vi "replace AO XYwfparam.vi"(0 "Baseline (V)":dbl, 1 "Start amplitude (V)":dbl, 2 "Cycles":dbl, 3 "Repeats":dbl, 4 "index of AO wave":i32, 5 "Step size (V)":dbl, 7 "DC (%)":dbl, 9 "Sampling frequency (Hz)":dbl, 11 "Period (ms)":dbl, 12 "Cycle length (s)":dbl, 13 "Pulses":dbl, 14 "padding value":dbl, 15 "Matlab wave name":path) -> ()   [LabVIEW 2015]
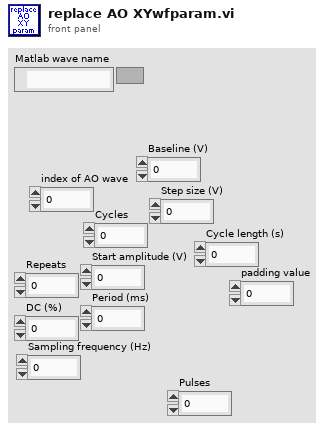
[diagram p1: front panel]
types:
  T1 = cluster{"AO parameters":cluster{"AOtab":dbl, "Repeats":dbl, "Cycles":dbl, "Start amplitude (V)":dbl, "Baseline (V)":dbl, "Step size (V)":dbl, "DC (%)":dbl, "Sampling frequency (Hz)":dbl, "Period (ms)":dbl, "Offset (V)":dbl, "Amplitude (V)":dbl, "Frequency":dbl, "Tri Repeats":dbl, "phase shift (ms)":dbl, "Pulses":dbl, "Matlab wave file":path, "Tri phase":dbl, "padding value":dbl}[], "DO parameters":cluster{"Digital DC (%)":dbl, "Digital phase":dbl, "Digital Freq (Hz)":dbl, "Sampling frequency (Hz)":dbl, "Digital time offset (s) ":dbl, "padding value":dbl, "matlab wave file":path, "DOtab":dbl}[]}
  T2 = cluster{"AOtab":dbl, "Repeats":dbl, "Cycles":dbl, "Start amplitude (V)":dbl, "Baseline (V)":dbl, "Step size (V)":dbl, "DC (%)":dbl, "Sampling frequency (Hz)":dbl, "Period (ms)":dbl, "Offset (V)":dbl, "Amplitude (V)":dbl, "Frequency":dbl, "Tri Repeats":dbl, "phase shift (ms)":dbl, "Pulses":dbl, "Matlab wave file":path, "Tri phase":dbl, "padding value":dbl}[]
  T3 = cluster{"AOtab":dbl, "Repeats":dbl, "Cycles":dbl, "Start amplitude (V)":dbl, "Baseline (V)":dbl, "Step size (V)":dbl, "DC (%)":dbl, "Sampling frequency (Hz)":dbl, "Period (ms)":dbl, "Offset (V)":dbl, "Amplitude (V)":dbl, "Frequency":dbl, "Tri Repeats":dbl, "phase shift (ms)":dbl, "Pulses":dbl, "Matlab wave file":path, "Tri phase":dbl, "padding value":dbl}
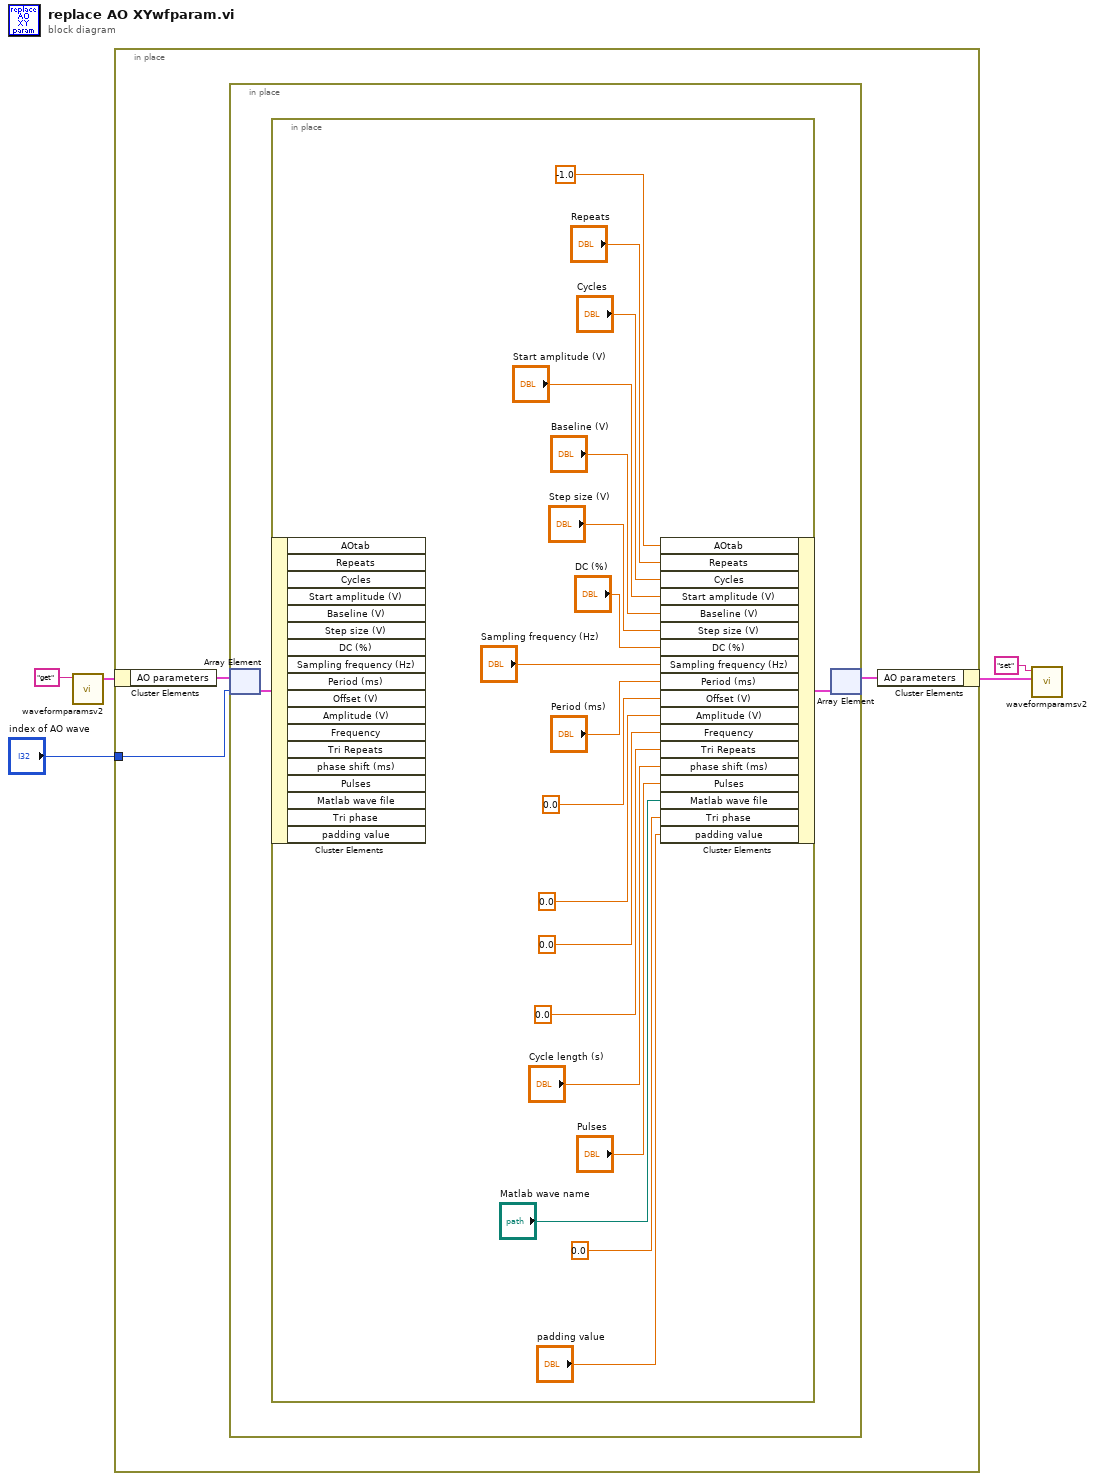
[diagram p0: block diagram]
diagram:
  n1 = call "waveformparamsv2.vi"("command"="get") -> ("Params out"=w3:T1)  [unwired: 4 in, 2 out]
  n2 = in-place {
    in-place-border: "index of AO wave" -> [w6]
    n3 = in-place-cluster #1(w3) -> ("AO parameters"=w8:T2)
    n4 = in-place {
      n5 = in-place-array #2(w8, w6) -> (w10:T3)
      n6 = in-place {
        n7 = in-place-cluster #3(w10) -> ()  [unwired: 18 out]
        n8 = in-place-cluster #3("AOtab"=-1.0, "Repeats"="Repeats", "Cycles"="Cycles", "Start amplitude (V)"="Start amplitude (V)", "Baseline (V)"="Baseline (V)", "Step size (V)"="Step size (V)", "DC (%)"="DC (%)", "Sampling frequency (Hz)"="Sampling frequency (Hz)", "Period (ms)"="Period (ms)", "Offset (V)"=0.0, "Amplitude (V)"=0.0, "Frequency"=0.0, "Tri Repeats"=0.0, "phase shift (ms)"="Cycle length (s)", "Pulses"="Pulses", "Matlab wave file"="Matlab wave name", "Tri phase"=0.0, "padding value"="padding value") -> (w9:T3)
      }
      n9 = in-place-array #2(w9) -> (w7:T2)  [unwired: 1 out]
    }
    n10 = in-place-cluster #1("AO parameters"=w7) -> (w4:T1)
  }
  n11 = call "waveformparamsv2.vi"("command"="set", "Params in"=w4) -> ()  [unwired: 3 in, 3 out]
